vi "MainGUI.vi"(0 "reference in":refnum<class "VerticalButtonBar.lvclass">, 5 "Error In":errorcluster) -> (14 "reference out":refnum<class "VerticalButtonBar.lvclass">, 19 "Error Out":errorcluster)   [LabVIEW 2021, in "VerticalButtonBar.lvclass"]
doc: "This is the user interface of the object. It will handle the events to update the GUI."
uses:
  VerticalButtonBar.lvclass
  VerticalButtonBar_MessageData.ctl
  ButtonCollection/ButtonCollection.lvclass
  4dc8a6fc-d3e0-427f-b90e-208f30f82a79.vi
  <vilib>/TriekselSoft/TracerLibrary/TracerLibrary/Tracer/protected/SendMessage.vi
  <vilib>/TriekselSoft/TracerLibrary/TracerLibrary/Tracer/protected/Timestamp.vi
  4dc8a6fc-d3e0-427f-b90e-208f30f82a79.vi/f75db090-0877-4668-94fb-75c2140b1617.vi
  <vilib>/TriekselSoft/TracerLibrary/TracerLibrary/Tracer/Tracer_Level-Info.vi
  <vilib>/JDP Science/JSONtext/Variant to JSON Text.vi
  <vilib>/TriekselSoft/TracerLibrary/TracerLibrary/Tracer/protected/Tracer_ClassAttributes.vi
  <vilib>/JDP Science/JSONtext/LVClass Serializer/JSONtext LVClass Serializer.lvclass
  VerticalButtonBar.lvclass/VerticalButtonBar.ctl
panel:
  in  "btn 1":bool
  out "Last Command":string
  in  "btn 2":bool
  in  "btn 3":bool
  in  "btn 4":bool
  in  "btn 5":bool
  in  "btn 6":bool
  in  "btn 7":bool
  in  "btn 8":bool
  in  "btn 9":bool
  in  "btn 10":bool
  in  "btn 11":bool
  in  "btn 12":bool
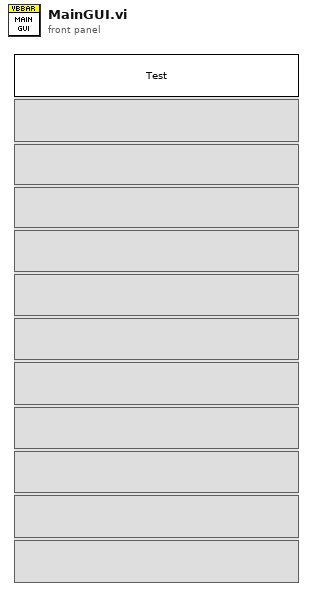
[diagram p1: front panel]
types:
  T1 = typedef "VerticalButtonBar.lvclass/VerticalButtonBar_MessageData.ctl" = cluster{"ShowWindow":cluster{"Send":cluster{"Show":bool}, "Receive":cluster{"Dummy":bool}}}
  T2 = cluster{"Event":refnum<event-registration>, "Command":string, "MessageData":T1, "ReplyQueue":refnum<queue>}
  T3 = cluster{"ReplyQueue":refnum<queue>, "Data":variant}
  T4 = typedef "ButtonCollection.lvclass/ButtonDefinition.ctl" = cluster{"ThisNavigationName":string, "ButtonLabel":string, "Caption":string, "Tooltip":string, "EnabledExpression":string, "Actions":cluster{"ActionType":string, "TargetObject":string, "Parameter":string, "WaitUntilDone":bool}[], "NextNavigationName":string}
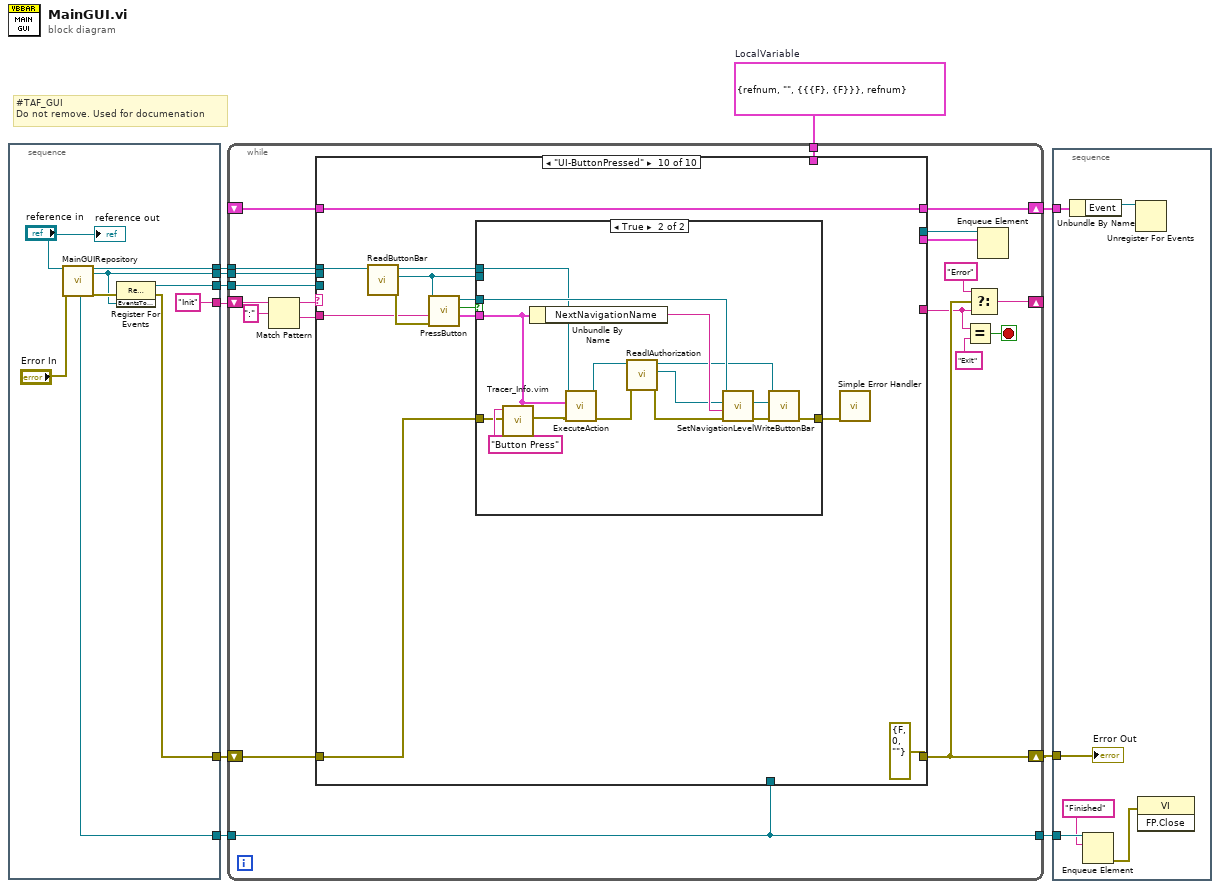
[diagram p0: block diagram]
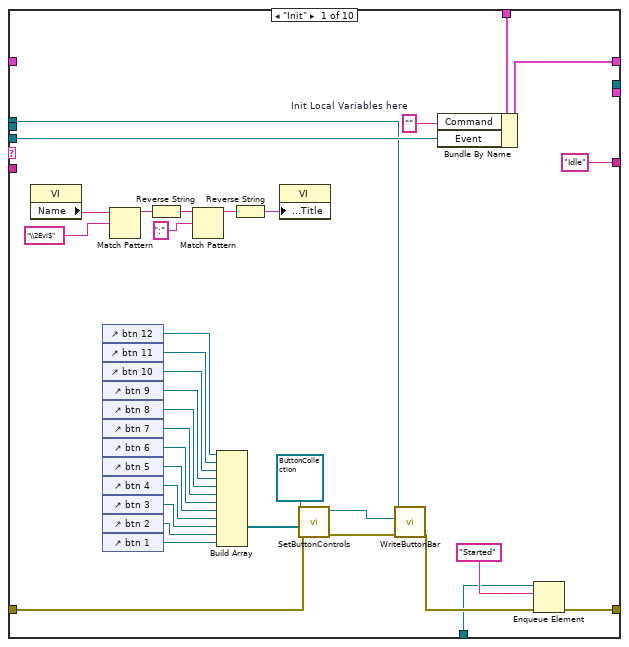
[diagram p2: hidden frame]
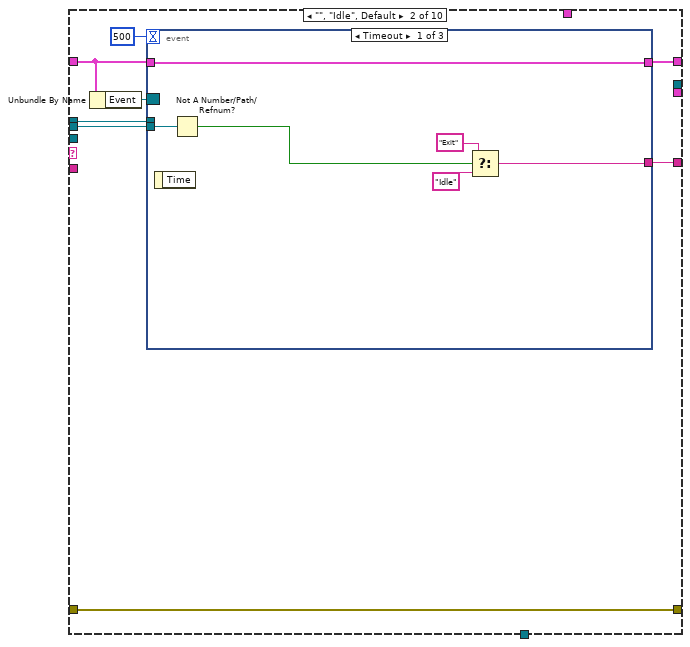
[diagram p3: hidden frame]
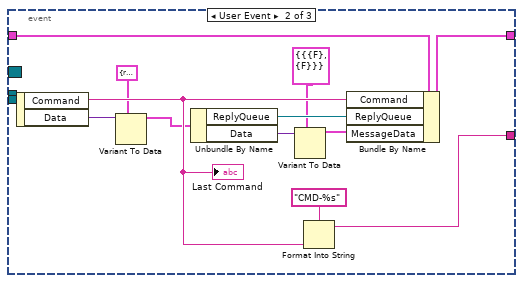
[diagram p4: hidden frame]
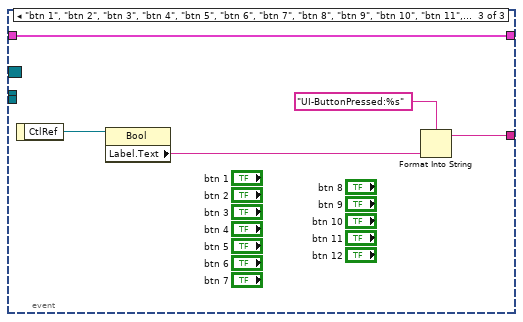
[diagram p5: hidden frame]
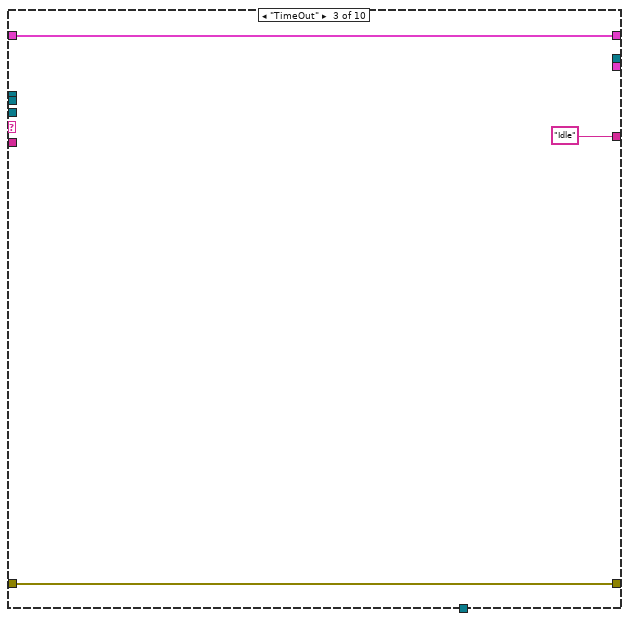
[diagram p6: hidden frame]
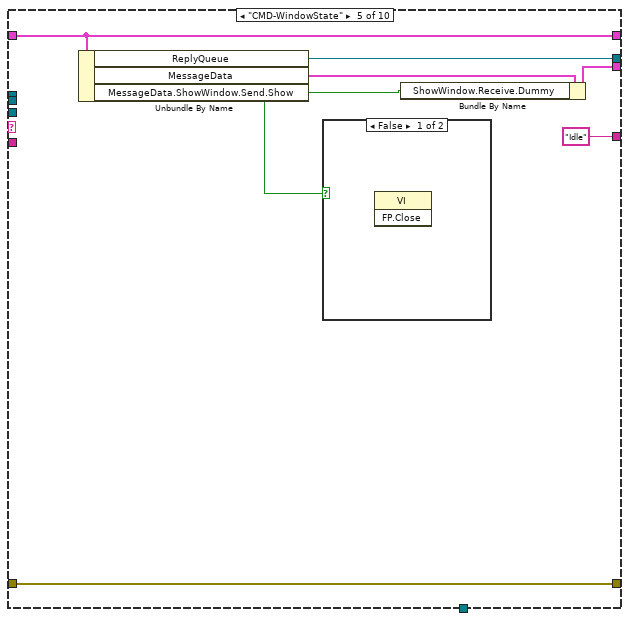
[diagram p8: hidden frame]
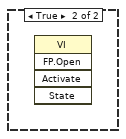
[diagram p9: hidden frame]
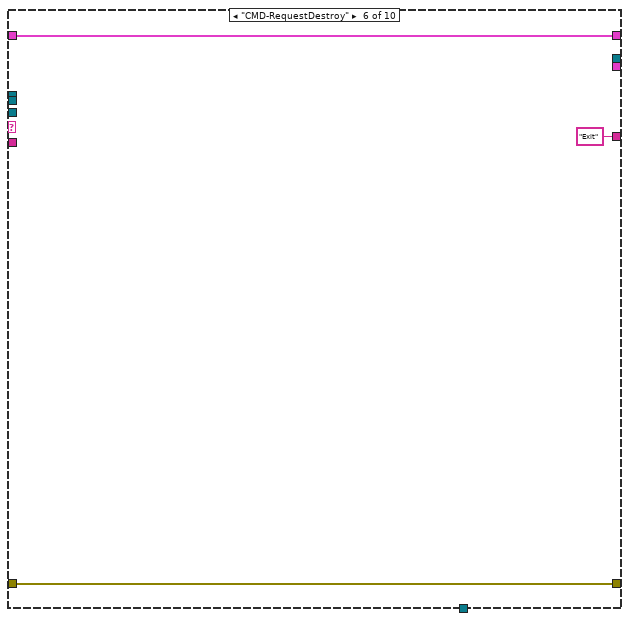
[diagram p10: hidden frame]
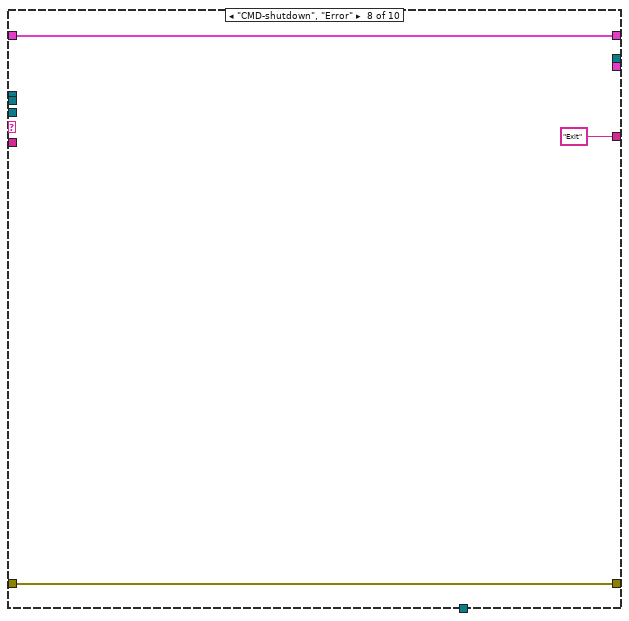
[diagram p12: hidden frame]
diagram:
  w5 = T2 {"Event"=refnum, "Command"="", "MessageData"={"ShowWindow"={"Send"={"Show"=FALSE}, "Receive"={"Dummy"=FALSE}}}, "ReplyQueue"=refnum}  # LocalVariable
  # "#TAF_GUI\nDo not remove. Used for documenation"
  n1 = stacked-sequence {
    tunnel: [w12] -> w10
    tunnel: [w19] -> w8
    tunnel: [w15] -> w7
    tunnel: ["Init"] -> w6
    tunnel: [w13] -> w3
    tunnel: [w11] -> w1
    frame #0 {
      n2 = call "MainGUIRepository.vi"("ReferenceIn"="reference in", "ErrorIn"="Error In") -> ("ProcessSyncQueue"=w13:refnum<queue>, "ReferenceOut"=w19:refnum<class "VerticalButtonBar.lvclass">, "EventsToProcess"=w11:refnum<user-event>, "ErrorOut"=w14:errorcluster)  [unwired: 10 in, 4 out]
      n3 = register-events(error in=w14, w11) -> (reference out=w15:refnum<event-registration>, error out=w12:errorcluster)  [unwired: 1 in]
      "reference out" <- "reference in"
    }
  }
  n4 = while {
    shift-right: [w32] -> w9
    shift-left: w10 -> [w37]
    tunnel: w8 -> [w38]
    tunnel: w7 -> [w39]
    shift-right: [w30] -> _
    shift-left: w6 -> [w35]
    shift-right: [w26] -> w4
    shift-left: _ -> [w25]
    tunnel: w5 -> [w24]
    tunnel: [w21] -> w2
    tunnel: w3 -> [w21]
    tunnel: w1 -> [w20]
    stop <- w27 stop-if-true
    n5 = Match Pattern(string=w35, regular expression=":") -> (before substring=w34:string, after substring=w33:string)  [unwired: 1 in, 2 out]
    n6 = case shown="\"UI-ButtonPressed\"" w34 {
      tunnel: w37 -> [w47 w76 w107 w109 w116 w119 w121 w124 w126 w132]
      tunnel: [w43 w76 w107 w109 w116 w119 w121 w124 w126 errorcluster {"status"=FALSE, "code"=0, "source"=""} ("error out")] -> w32
      tunnel: w39 -> [w62 _ _ _ _ _ _ _ _ _]
      tunnel: w38 -> [w46 w75 _ _ _ _ _ _ _ w137]
      tunnel: w33 -> [_ _ _ _ _ _ _ _ _ w135]
      tunnel: ["Idle" ("t") w81 "Idle" ("t") _ "Idle" ("t") "Exit" ("y") _ "Exit" ("y") _ _] -> w29
      tunnel: [w73 w80 w105 w108 w114 w118 w120 w122 w125 w138] -> w26
      tunnel: w25 -> [_ w79 w105 w108 w114 w118 w120 w122 w125 w138]
      tunnel: w24 -> [w70 _ _ _ _ _ _ _ _ _]
      tunnel: [_ _ _ _ w113 _ _ _ _ _] -> w23
      tunnel: [_ _ _ _ w111 _ _ _ _ _] -> w22
      tunnel: w21 -> [w42 _ _ _ _ _ _ _ _ _]
      tunnel: w20 -> [_ w74 _ _ _ _ _ _ _ _]
      frame "Init" {
        w72 = ""  # Init Local Variables here
        n7 = property class="VI"() -> ("Name"=w69:string)  [unwired: 2 in, 2 out]
        n8 = control-ref of="btn 12"() -> (w50:refnum<vi>)
        n9 = control-ref of="btn 11"() -> (w51:refnum<vi>)
        n10 = control-ref of="btn 10"() -> (w52:refnum<vi>)
        n11 = control-ref of="btn 9"() -> (w53:refnum<vi>)
        n12 = control-ref of="btn 8"() -> (w54:refnum<vi>)
        n13 = control-ref of="btn 7"() -> (w55:refnum<vi>)
        n14 = control-ref of="btn 6"() -> (w56:refnum<vi>)
        n15 = control-ref of="btn 5"() -> (w57:refnum<vi>)
        n16 = control-ref of="btn 4"() -> (w58:refnum<vi>)
        n17 = control-ref of="btn 3"() -> (w59:refnum<vi>)
        n18 = control-ref of="btn 2"() -> (w60:refnum<vi>)
        n19 = control-ref of="btn 1"() -> (w61:refnum<vi>)
        n20 = Match Pattern(string=w69, regular expression="\\2Evi$") -> (before substring=w67:string)  [unwired: 1 in, 3 out]
        n21 = Reverse String(1:w67) -> (0:w66:string)
        n22 = Match Pattern(string=w66, regular expression=":") -> (before substring=w64:string)  [unwired: 1 in, 3 out]
        n23 = Build Array(w50, w51, w52, w53, w54, w55, w56, w57, w58, w59, w60, w61) -> (w48:refnum<vi>[])
        n24 = Reverse String(1:w64) -> (0:w63:string)
        n25 = property class="VI"("Front Panel.Title"=w63) -> ()  [unwired: 2 in, 2 out]
        n26 = call-dynamic "SetButtonControls.vi"("ErrorIn"=w47, "Buttons"=w48, "ObjectIn"=refnum<class "ButtonCollection.lvclass"> refnum ("ButtonCollection")) -> ("ErrorOut"=w41:errorcluster, "ObjectOut"=w40:refnum<class "ButtonCollection.lvclass">)  [unwired: 7 in]
        n27 = call-dynamic "WriteButtonBar.vi"("ErrorIn"=w41, "ButtonBar"=w40, "ReferenceIn"=w46) -> ("ErrorOut"=w44:errorcluster)  [unwired: 7 in, 1 out]
        n28 = Bundle By Name(cluster=w70, "Command"=w72, "Event"=w62) -> (w73:T2)
        n29 = Enqueue Element(queue=w42, element="Started", error in (no error)=w44) -> (error out=w43:errorcluster)  [unwired: 1 in, 2 out]
      }
      frame "", "Idle", Default {
        n30 = Unbundle By Name(w79) -> ("Event"=w78:refnum<event-registration>)
        n31 = event shown="[0] Timeout" {
          selector: w78 -> [_ _ _]
          dyn-events: _ -> [_ _ _]
          timeout: 500 -> [_ _ _]
          tunnel: [w84 w96 w100] -> w81
          tunnel: w79 -> [w87 w99 w104]
          tunnel: [w87 w98 w104] -> w80
          tunnel: w75 -> [_ _ _]
          tunnel: w74 -> [w83 _ _]
          event Timeout {
            n32 = event-data() -> ()  [unwired: 1 in, 1 out]
            n33 = Not A Number/Path/Refnum?(number/path/refnum=w83) -> (NaN/Path/Refnum?=w82:bool)
            n34 = Select(t="Exit", s=w82, f="Idle" ("t")) -> (s? t:f=w84:string)
          }
          event User Event {
            n35 = event-data() -> ("Command"=w95:string, "Data"=w94:variant)  [unwired: 1 in]
            "Last Command" <- w95
            n36 = Variant To Data(type=T3 {"ReplyQueue"=refnum, "Data"=variant} ("output cluster"), Variant=w94) -> (data=w92:T3)  [unwired: 1 in, 1 out]
            n37 = Unbundle By Name(w92) -> ("ReplyQueue"=w91:refnum<queue>, "Data"=w90:variant)
            n38 = Variant To Data(type=T1 {"ShowWindow"={"Send"={"Show"=FALSE}, "Receive"={"Dummy"=FALSE}}} ("MessageData"), Variant=w90) -> (data=w89:T1)  [unwired: 1 in, 1 out]
            n39 = Format Into String(format string="CMD-%s", w95) -> (resulting string=w96:string)  [unwired: 2 in, 1 out]
            n40 = Bundle By Name(cluster=w99, "Command"=w95, "ReplyQueue"=w91, "MessageData"=w89) -> (w98:T2)
          }
          event "btn 1", "btn 2", "btn 3", "btn 4", "btn 5", "btn 6", "btn 7", "btn 8", "btn 9", "btn 10", "btn 11", "btn 12": Value Change {
            n41 = event-data() -> ("CtlRef"=w103:refnum<vi>)  [unwired: 1 in]
            n42 = property class="Bool"(reference=w103) -> ("Label.Text"=w101:string)  [unwired: 1 in, 2 out]
            n43 = Format Into String(format string="UI-ButtonPressed:%s", w101) -> (resulting string=w100:string)  [unwired: 2 in, 1 out]
          }
        }
      }
      frame "TimeOut" {
      }
      frame "---- COMMANDS START----" {
      }
      frame "CMD-WindowState" {
        n44 = Unbundle By Name(w114) -> ("ReplyQueue"=w113:refnum<queue>, "MessageData"=w112:T1, "MessageData.ShowWindow.Send.Show"=w110:bool)
        n45 = case shown="False" w110 {
          frame False {
            n46 = invoke class="VI" method="FP.Close"() -> ()  [unwired: 3 in, 3 out]
          }
          frame True {
            n47 = invoke class="VI" method="FP.Open"() -> ()  [unwired: 5 in, 5 out]
          }
        }
        n48 = Bundle By Name(cluster=w112, "ShowWindow.Receive.Dummy"=w110) -> (w111:T1)
      }
      frame "CMD-RequestDestroy" {
      }
      frame "----- COMMANDS END ----" {
      }
      frame "CMD-shutdown", "Error" {
      }
      frame "----- UI ACTIONS -----" {
      }
      frame "UI-ButtonPressed" {
        n49 = call-dynamic "ReadButtonBar.vi"("ReferenceIn"=w137) -> ("ErrorOut"=w136:errorcluster, "ButtonBar"=w130:refnum<class "ButtonCollection.lvclass">, "ReferenceIn"=w129:refnum<class "VerticalButtonBar.lvclass">)  [unwired: 8 in]
        n50 = call-dynamic "PressButton.vi"("ErrorIn"=w136, "Button"=w135, "ObjectIn"=w130) -> ("SelectedButton"=w133:T4, "Valid"=w134:bool, "ObjectOut"=w131:refnum<class "ButtonCollection.lvclass">)  [unwired: 5 in, 1 out]
        n51 = case shown="True" w134 {
          tunnel: w133 -> [_ w148]
          tunnel: [w139 w150] -> w127
          tunnel: w132 -> [w139 w147]
          tunnel: w131 -> [_ w153]
          tunnel: w130 -> [_ _]
          tunnel: w129 -> [_ w145]
          frame False {
          }
          frame True {
            n52 = call "Tracer_Info.vim"("Data"=w148, "Error In"=w147, "Info Text"="Button Press" ("InfoText")) -> ("Error Out"=w146:errorcluster)  [unwired: 8 in]
            n53 = Unbundle By Name(w148) -> ("NextNavigationName"=w154:string)
            n54 = call "ExecuteAction.vi"("ErrorIn"=w146, "ButtonDefinition"=w148, "VerticalButtonBarIn"=w145) -> ("ErrorOut"=w141:errorcluster, "VerticalButtonBarOut"=w140:refnum<class "VerticalButtonBar.lvclass">)  [unwired: 7 in]
            n55 = call-dynamic "ReadIAuthorization.vi"("ErrorIn"=w141, "ReferenceIn"=w140) -> ("ErrorOut"=w142:errorcluster, "IAuthorization"=w143:refnum<class "IAuthorization.lvclass">, "ReferenceIn"=w144:refnum<class "VerticalButtonBar.lvclass">)  [unwired: 7 in]
            n56 = call-dynamic "SetNavigationLevel.vi"("ErrorIn"=w142, "NavigationName"=w154, "Authorization"=w143, "ObjectIn"=w153) -> ("ErrorOut"=w151:errorcluster, "ObjectOut"=w152:refnum<class "ButtonCollection.lvclass">)  [unwired: 6 in]
            n57 = call-dynamic "WriteButtonBar.vi"("ErrorIn"=w151, "ButtonBar"=w152, "ReferenceIn"=w144) -> ("ErrorOut"=w150:errorcluster)  [unwired: 7 in, 1 out]
          }
        }
        n58 = call <vilib>:"Simple Error Handler.vi"("error in (no error)"=w127) -> ()  [unwired: 4 in, 5 out]
      }
    }
    n59 = Equal?(x=w29, y="Exit") -> (x = y?=w27:bool)
    n60 = Select(t="Error", s=w32, f=w29) -> (s? t:f=w30:string)
    n61 = Enqueue Element(queue=w23, element=w22) -> ()  [unwired: 2 in, 3 out]
  }
  n62 = stacked-sequence {
    tunnel: w9 -> [w160]
    tunnel: w2 -> [w157]
    tunnel: w4 -> [w159]
    frame #0 {
      n63 = Unbundle By Name(w159) -> ("Event"=w158:refnum<event-registration>)
      n64 = Enqueue Element(queue=w157, element="Finished") -> (error out=w156:errorcluster)  [unwired: 2 in, 2 out]
      n65 = Unregister For Events(event registration refnum=w158) -> ()  [unwired: 1 in, 1 out]
      n66 = invoke class="VI" method="FP.Close"(error in=w156) -> ()  [unwired: 2 in, 3 out]
      "Error Out" <- w160
    }
  }
